vi "Check Sections and Parameters (SubVI).vi"(8 "entrée d'erreur (pas d'erreur)":errorcluster, 9 "found? array":bool[][](array[boolean]), 10 "Parameter array":string[][](array[string]), 11 "Section array":string[](array[string])) -> (0 "sortie d'erreur":errorcluster, 3 "Erreur ?":bool)   [LabVIEW 2017]
doc: "by Tanguy BOULARD"
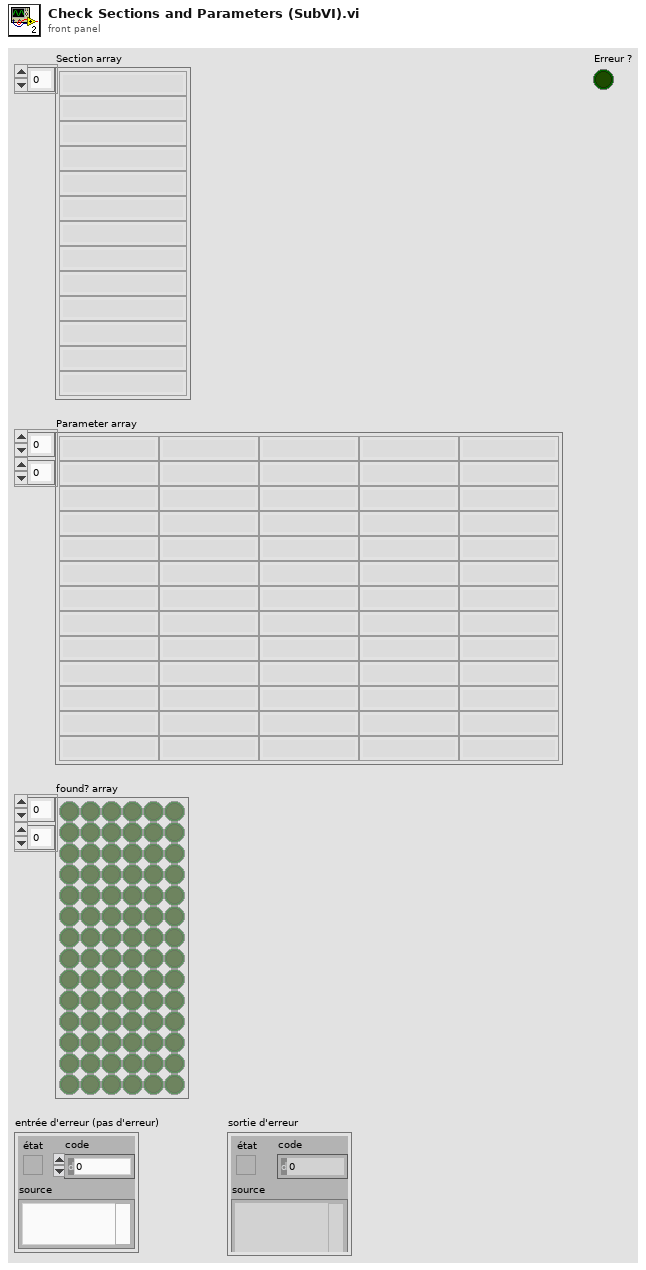
[diagram p1: front panel]
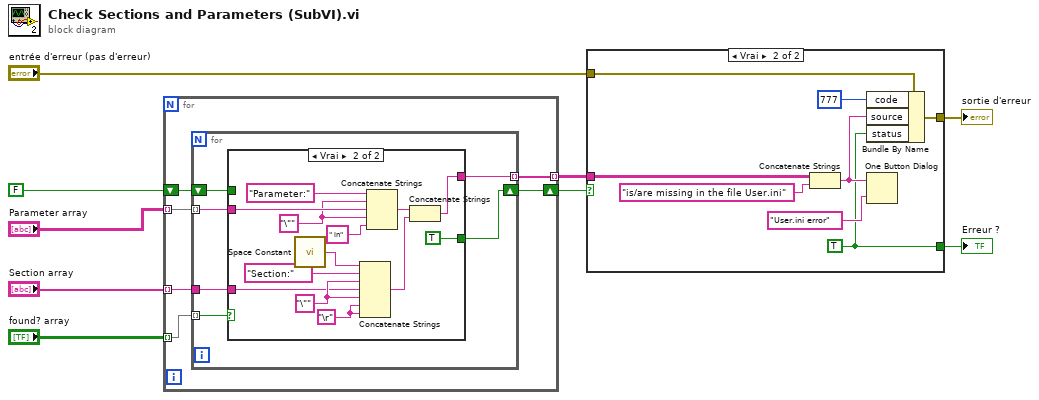
[diagram p0: block diagram]
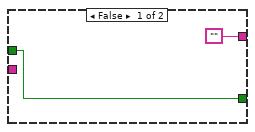
[diagram p2: hidden frame]
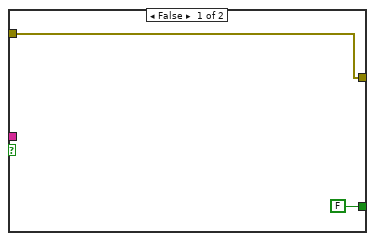
[diagram p3: hidden frame]
diagram:
  n1 = for {
    tunnel: [w15] -> w3 mode=indexing
    tunnel: "Section array" -> [w14] mode=indexing
    tunnel: "Parameter array" -> [w13] mode=indexing
    tunnel: "found? array" -> [w12] mode=indexing
    shift-right: [w11] -> w2
    shift-left: FALSE -> [w10]
    n2 = for {
      tunnel: w12 -> [w21] mode=indexing
      tunnel: w13 -> [w20] mode=indexing
      tunnel: [w19] -> w15 mode=indexing
      tunnel: w14 -> [w18]
      shift-right: [w17] -> w11
      shift-left: w10 -> [w16]
      n3 = case shown="Vrai" w21 {
        tunnel: w20 -> [_ w36]
        tunnel: ["" w30] -> w19
        tunnel: w18 -> [_ w33]
        tunnel: [w22 TRUE] -> w17
        tunnel: w16 -> [w22 _]
        frame False {
        }
        frame True {
          w24 = "\r"
          w34 = "\""
          w35 = "\""
          n4 = call <vilib>:"Space Constant.vi"() -> ("String"=w26:string)
          n5 = Concatenate Strings(w26, "Section:" ("Title"), w34, w33, w34, w24, w24) -> (w28:string)
          n6 = Concatenate Strings("Parameter:" ("Title"), w35, w36, w35, " in" ("string")) -> (w29:string)
          n7 = Concatenate Strings(w29, w28) -> (w30:string)
        }
      }
    }
  }
  n8 = case shown="Vrai" w2 {
    tunnel: w3 -> [_ w45]
    tunnel: [w38 w44] -> w7
    tunnel: "entrée d'erreur (pas d'erreur)" -> [w38 w43]
    tunnel: [FALSE ("status") w40] -> w9
    frame False {
    }
    frame True {
      w40 = TRUE ("status")
      n9 = Concatenate Strings(w45, "is/are missing in the file User.ini" ("Title")) -> (w42:string)
      n10 = Bundle By Name(cluster=w43, "code"=777, "source"=w42, "status"=w40) -> (w44:errorcluster)
      n11 = One Button Dialog(message=w42, button name ("OK")="User.ini error" ("Title")) -> ()  [unwired: 1 out]
    }
  }
  "sortie d'erreur" <- w7
  "Erreur ?" <- w9
